vi "rad_Configure Target.vi"(5 "Password":string, 8 "error in (no error)":errorcluster, 9 "Target settings in":T1={"Hostname"="", "Serial number"="", "Product name"="", "Product code"=0, "System status"="", "Credential type"=enum."None/Unlocked", "User added?"=FALSE, "Primary NIC"={"MAC address"="", "IP Address Request Mode"=2, "IP address"="", "Subnet mask"="", "Gateway"="", "DNS server"=""}} {"Primary NIC"."IP Address Request Mode" items=["Static"=1, "DHCP/Link-Local"=2, "Link-Local Only"=4, "DHCP Only"=8]}, 11 "Target Config Options in":T3={"NumInBatch"=0, "Target Config Operation"=enum."No Config", "Target Name"="", "Increment Static IPs"=FALSE, "Change Target Name"=FALSE, "Primary NIC"={"MAC address"="", "IP Address Request Mode"=2, "IP address"="", "Subnet mask"="", "Gateway"="", "DNS server"=""}} {"Primary NIC"."IP Address Request Mode" items=["Static"=1, "DHCP/Link-Local"=2, "Link-Local Only"=4, "DHCP Only"=8]}) -> (0 "error out":errorcluster, 1 "Target settings out":T1={"Hostname"="", "Serial number"="", "Product name"="", "Product code"=0, "System status"="", "Credential type"=enum."None/Unlocked", "User added?"=FALSE, "Primary NIC"={"MAC address"="", "IP Address Request Mode"=2, "IP address"="", "Subnet mask"="", "Gateway"="", "DNS server"=""}} {"Primary NIC"."IP Address Request Mode" items=["Static"=1, "DHCP/Link-Local"=2, "Link-Local Only"=4, "DHCP Only"=8]}, 3 "Target Config Options out":T3={"NumInBatch"=0, "Target Config Operation"=enum."No Config", "Target Name"="", "Increment Static IPs"=FALSE, "Change Target Name"=FALSE, "Primary NIC"={"MAC address"="", "IP Address Request Mode"=2, "IP address"="", "Subnet mask"="", "Gateway"="", "DNS server"=""}} {"Primary NIC"."IP Address Request Mode" items=["Static"=1, "DHCP/Link-Local"=2, "Link-Local Only"=4, "DHCP Only"=8]})   [LabVIEW 2020]
uses:
  App Images/TypeDefs/rad_Target Configuration Operations.ctl
  TypeDefs/rad_Target Network Settings.ctl
  App Images/TypeDefs/rad_Target Configuration Settings.ctl
  TypeDefs/rad_Target Information.ctl
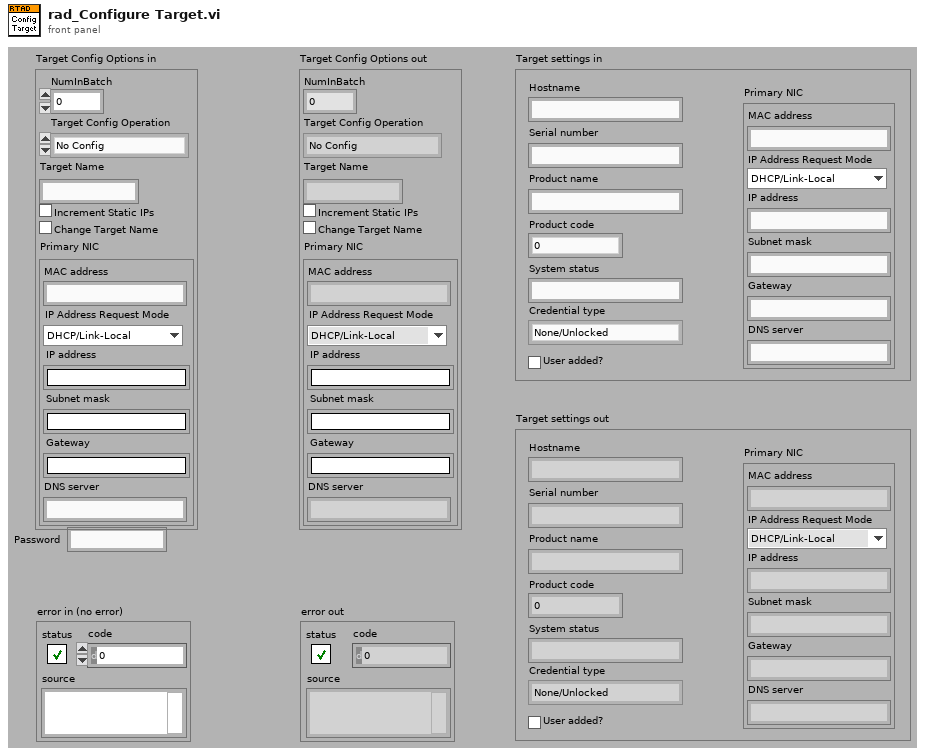
[diagram p1: front panel]
types:
  T1 = typedef "rad_Target Information.ctl" = cluster{"Hostname":string, "Serial number":string, "Product name":string, "Product code":i32, "System status":string, "Credential type":enum16{"None/Unlocked", "FTP Password", "NIAuth Credentials"}, "User added?":bool, "Primary NIC":T2}
  T2 = typedef "rad_Target Network Settings.ctl" = cluster{"MAC address":string, "IP Address Request Mode":i32, "IP address":string, "Subnet mask":string, "Gateway":string, "DNS server":string}
  T3 = typedef "rad_Target Configuration Settings.ctl" = cluster{"NumInBatch":u32, "Target Config Operation":T4, "Target Name":string, "Increment Static IPs":bool, "Change Target Name":bool, "Primary NIC":T2}
  T4 = typedef "rad_Target Configuration Operations.ctl" = enum8{"No Config", "Image Config", "Static Config"}
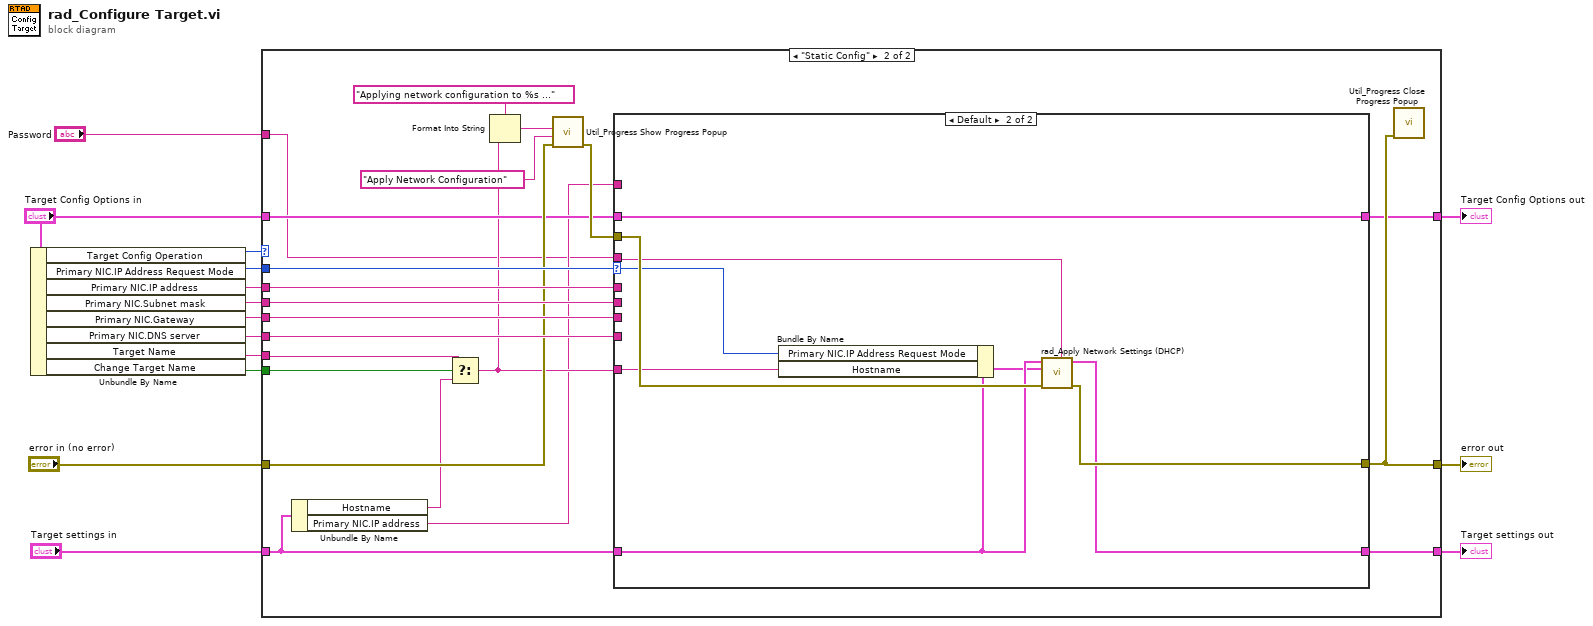
[diagram p0: block diagram]
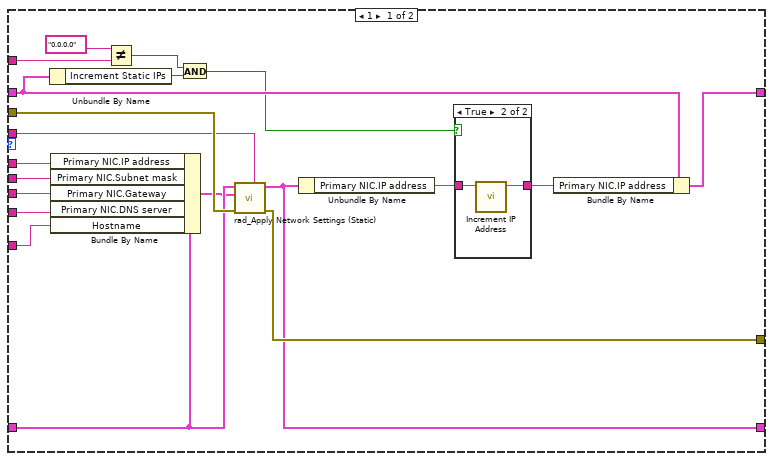
[diagram p3: hidden frame]
diagram:
  n1 = Unbundle By Name("Target Config Options in") -> ("Target Config Operation"=w15:T4, "Primary NIC.IP Address Request Mode"=w14:i32, "Primary NIC.IP address"=w13:string, "Primary NIC.Subnet mask"=w5:string, "Primary NIC.Gateway"=w12:string, "Primary NIC.DNS server"=w11:string, "Target Name"=w7:string, "Change Target Name"=w8:bool)
  n2 = case shown="\"Static Config\"" w15 {
    tunnel: w14 -> [_ w39]
    tunnel: w13 -> [_ w38]
    tunnel: w5 -> [_ w37]
    tunnel: w12 -> [_ w36]
    tunnel: w11 -> [_ w35]
    tunnel: "error in (no error)" -> [w18 w32]
    tunnel: [w18 w30] -> w9
    tunnel: w8 -> [_ w28]
    tunnel: w7 -> [_ w27]
    tunnel: "Target Config Options in" -> [w17 w26]
    tunnel: [w17 w25] -> w4
    tunnel: "Target settings in" -> [w16 w22]
    tunnel: [w16 w23] -> w2
    tunnel: "Password" -> [_ w19]
    frame Default {
    }
    frame "Static Config" {
      n3 = Unbundle By Name(w22) -> ("Hostname"=w20:string, "Primary NIC.IP address"=w21:string)
      n4 = Select(t=w27, s=w28, f=w20) -> (s? t:f=w24:string)
      n5 = Format Into String(format string="Applying network configuration to %s ..." ("Message"), w24) -> (resulting string=w33:string)  [unwired: 2 in, 1 out]
      n6 = call "Util_Progress Show Progress Popup.vi"("error in (no error)"=w32, "Title"="Apply Network Configuration", "Message"=w33) -> ("error out"=w29:errorcluster)  [unwired: 8 in]
      n7 = case shown="Default" w39 {
        selector: w39 -> [_ w64]
        tunnel: w38 -> [w59 _]
        tunnel: w37 -> [w58 _]
        tunnel: w36 -> [w57 _]
        tunnel: w35 -> [w56 _]
        tunnel: [w46 w71] -> w30
        tunnel: w29 -> [w55 w70]
        tunnel: w21 -> [w54 _]
        tunnel: w26 -> [w50 w69]
        tunnel: [w49 w69] -> w25
        tunnel: w24 -> [w47 w67]
        tunnel: w22 -> [w42 w66]
        tunnel: [w43 w68] -> w23
        tunnel: w19 -> [w40 w63]
        frame 1 {
          n8 = Unbundle By Name(w50) -> ("Increment Static IPs"=w52:bool)
          n9 = Bundle By Name(cluster=w42, "Primary NIC.IP address"=w59, "Primary NIC.Subnet mask"=w58, "Primary NIC.Gateway"=w57, "Primary NIC.DNS server"=w56, "Hostname"=w47) -> (w41:T1)
          n10 = Not Equal?(x="0.0.0.0" ("y"), y=w54) -> (x != y?=w51:bool)
          n11 = And(x=w51, y=w52) -> (x .and. y?=w48:bool)
          n12 = call "rad_Apply Network Settings (Static).vi"("Password"=w40, "error in (no error)"=w55, "Requested settings"=w41, "Existing settings"=w42) -> ("error out"=w46:errorcluster, "Target settings out"=w43:T1)  [unwired: 6 in]
          n13 = Unbundle By Name(w43) -> ("Primary NIC.IP address"=w44:string)
          n14 = case shown="True" w48 {
            tunnel: w44 -> [w60 w62]
            tunnel: [w60 w61] -> w45
            frame False {
            }
            frame True {
              n15 = call "Increment IP Address.vi"("IP Address"=w62) -> ("New IP Address"=w61:string)  [unwired: 8 in, 2 out]
            }
          }
          n16 = Bundle By Name(cluster=w50, "Primary NIC.IP address"=w45) -> (w49:T3)
        }
        frame Default {
          n17 = Bundle By Name(cluster=w66, "Primary NIC.IP Address Request Mode"=w64, "Hostname"=w67) -> (w65:T1)
          n18 = call "rad_Apply Network Settings (DHCP).vi"("Password"=w63, "error in (no error)"=w70, "Requested settings"=w65, "Existing settings"=w66) -> ("error out"=w71:errorcluster, "Target settings out"=w68:T1)  [unwired: 6 in]
        }
      }
      n19 = call "Util_Progress Close Progress Popup.vi"("error in (no error)"=w30) -> ()  [unwired: 10 in, 1 out]
    }
  }
  "error out" <- w9
  "Target Config Options out" <- w4
  "Target settings out" <- w2
